vi "Run Delayed Inject.vi"(8 "error in (no error)":errorcluster, 10 "Injection delay":dbl format="%#_g s", 11 "cetoni in":refnum<class "cetoni.lvclass">) -> (0 "error out":errorcluster, 3 "cetoni out":refnum<class "cetoni.lvclass">)   [LabVIEW 2018, in "cetoni.lvlib" / "cetoni.lvclass"]
uses:
  cetoni.lvclass
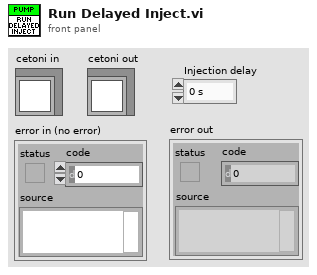
[diagram p1: front panel]
types:
  T1 = enum16{"LOW_PRESSURE_VALVE", "BALL_VALVE", "QMIX_VALVE"}
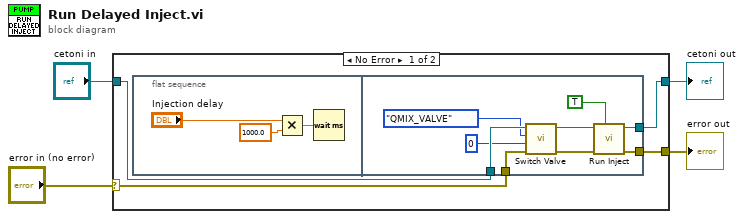
[diagram p0: block diagram]
diagram:
  n1 = case shown="No Error" "error in (no error)" {
    selector: "error in (no error)" -> [w8 w22]
    tunnel: [w7 w22] -> w3
    tunnel: [w6 w21] -> w1
    tunnel: "cetoni in" -> [w5 w21]
    frame No Error {
      n2 = flat-sequence {
        tunnel: w5 -> [w15]
        tunnel: w8 -> [w14]
        tunnel: [w19] -> w7
        tunnel: [w18] -> w6
        frame #0 {
          n3 = Multiply(x="Injection delay", y=1000.0) -> (x*y=w9:dbl)
          n4 = Wait (ms)(milliseconds to wait=w9) -> ()  [unwired: 1 out]
        }
        frame #1 {
          n5 = call-dynamic "Switch Valve.vi"("error in (no error)"=w14, "pos"=0, "valve"=T1."QMIX_VALVE", "PHD Ultra in"=w15) -> ("error out"=w16:errorcluster, "PHD Ultra out"=w17:refnum<class "cetoni.lvclass">)  [unwired: 6 in]
          n6 = call-dynamic "Run Inject.vi"("auto_switch_valve"=TRUE, "error in (no error)"=w16, "PHD Ultra in"=w17) -> ("error out"=w19:errorcluster, "PHD Ultra out"=w18:refnum<class "cetoni.lvclass">)  [unwired: 7 in]
        }
      }
    }
    frame Error {
    }
  }
  "error out" <- w3
  "cetoni out" <- w1
